vi "LVRT Serial Read LIDAR.vi"(6 "Termination Character (Linefeed)":string="\n", 8 "error in (no error)":errorcluster, 9 "Timeout (ms) (-1: no timeout)":i32=-1, 10 "Bytes to Read":u32, 11 "FPGA Main Ref":T1) -> (0 "error out":errorcluster, 2 "LIDAR":string, 3 "FPGA Main Ref Out":T1)   [LabVIEW 2010]
uses:
  <vilib>/rvi/interface/nirviReadWriteControl/nirviReadWriteControl.xnode
  serial FPGA Main.vi
  FPGA Bitfiles/Athena Brain.lvproj_FPGA Target 2_serial FPGA Main.vi.lvbitx
  serial FPGA main reference type def.ctl
  <vilib>/rvi/errors/niLvFpgaWhatHappensToTopLevelVI.ctl
  <vilib>/rvi/interface/common/niFpgaNodeNameForErrorReporting.ctl
  <vilib>/rvi/errors/niLvFpgaAdjustHostInterfaceError.vi
  <vilib>/RVI Host/nirviSupport.llb/nirviErrorClusterFromErrorCode.vi
panel:
  out "Bytes read so far":u32
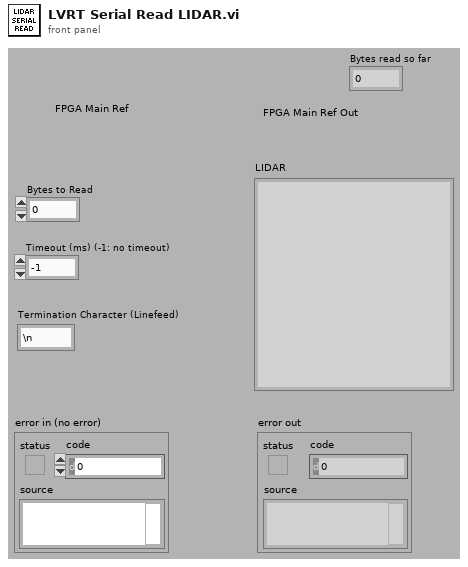
[diagram p1: front panel]
types:
  T1 = typedef "serial FPGA main reference type def.ctl" = refnum<k20>
  T2 = typedef "niFpgaNodeNameForErrorReporting.ctl" = enum16{"Open FPGA VI Reference", "Read/Write Control", "Invoke Method: Abort", "Invoke Method: Acknowledge IRQ", "Invoke Method: Download", "Invoke Method: FIFO.Configure", "Invoke Method: FIFO.Read", "Invoke Method: FIFO.Start", "Invoke Method: FIFO.Stop", "Invoke Method: FIFO.Write", "Invoke Method: Reset", "Invoke Method: Run", "Invoke Method: Wait on IRQ", "Close FPGA VI Reference"}
  T3 = typedef "niLvFpgaWhatHappensToTopLevelVI.ctl" = enum16{"top level VI scripted behind XNode", "top level VI inlined behind XNode"}
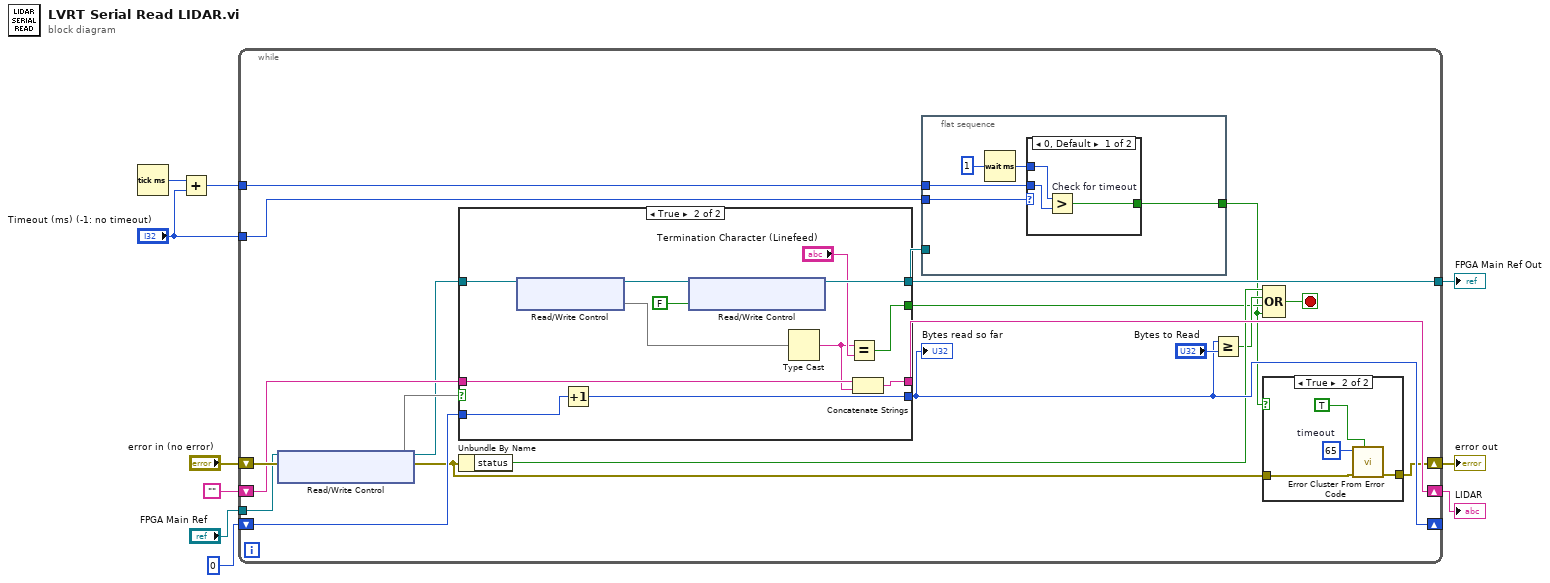
[diagram p0: block diagram]
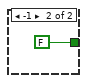
[diagram p3: hidden frame]
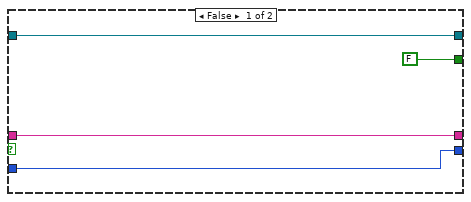
[diagram p4: hidden frame]
diagram:
  n1 = Tick Count (ms)() -> (millisecond timer value=w3:u32)
  n2 = Add(x=w3, y="Timeout (ms) (-1: no timeout)") -> (x+y=w1:u32)
  n3 = while {
    tunnel: "FPGA Main Ref" -> [w23]
    tunnel: [w21] -> w7
    shift-right: [w20] -> _
    shift-left: u32 0 -> [w27]
    shift-right: [w25] -> w4
    shift-left: "" -> [w26]
    shift-right: [w11] -> w9
    shift-left: "error in (no error)" -> [w29]
    tunnel: "Timeout (ms) (-1: no timeout)" -> [w15]
    tunnel: w1 -> [w14]
    stop <- w17 stop-if-true
    n4 = xnode "Read/Write Control"("FPGA VI Reference In"=w23, "error in"=w29) -> ("FPGA VI Reference Out"=w22:T1, "error out"=w12:errorcluster, "LIDAR Read: New Data"=w28)
    n5 = case shown="True" w28 {
      tunnel: [w47 w59] -> w20
      tunnel: w27 -> [w47 w58]
      tunnel: w26 -> [w46 w57]
      tunnel: [w46 w56] -> w25
      tunnel: w22 -> [w45 w54]
      tunnel: [w45 w52] -> w21
      tunnel: [FALSE w49] -> w16
      frame False {
      }
      frame True {
        n6 = xnode "Read/Write Control"("FPGA VI Reference In"=w54) -> ("FPGA VI Reference Out"=w53:T1, "LIDARRead: Char"=w55)  [unwired: 1 in, 1 out]
        n7 = Increment(x=w58) -> (x+1=w59:u32)
        n8 = xnode "Read/Write Control"("FPGA VI Reference In"=w53, "LIDAR Read: New Data"=FALSE ("Data Read")) -> ("FPGA VI Reference Out"=w52:T1)  [unwired: 1 in, 1 out]
        n9 = Type Cast(x=w55) -> (*(type *) &x=w50:string)  [unwired: 1 out]
        n10 = Equal?(x=w50, y="Termination Character (Linefeed)") -> (x = y?=w49:bool)
        n11 = Concatenate Strings(w57, w50) -> (w56:string)
      }
    }
    "Bytes read so far" <- w20
    n12 = Unbundle By Name(w12) -> ("status"=w19:bool)
    n13 = flat-sequence {
      tunnel: w21 -> [_]
      tunnel: [w38] -> w13
      tunnel: w15 -> [w37]
      tunnel: w14 -> [w36]
      frame #0 {
        n14 = Wait (ms)(milliseconds to wait=u32 1) -> (millisecond timer value=w35:u32)
        n15 = case shown="0, Default" w37 {
          tunnel: [w40 FALSE] -> w38
          tunnel: w36 -> [w41 _]
          tunnel: w35 -> [w42 _]
          frame 0, Default {
            n16 = Greater? "Check for timeout"(x=w42, y=w41) -> (0:w40:bool)
          }
          frame -1 {
          }
        }
      }
    }
    n17 = Greater Or Equal?(x=w20, y="Bytes to Read") -> (x >= y?=w18:bool)
    n18 = Compound Arithmetic op=OR(w19, w18, w16, w13) -> (w17:bool)
    n19 = case shown="True" w13 {
      tunnel: w12 -> [w30 w34]
      tunnel: [w30 w33] -> w11
      frame False {
      }
      frame True {
        w32 = 65  # timeout
        n20 = call <vilib>:"Error Cluster From Error Code.vi"("show call chain? (False)"=TRUE, "error in (no error)"=w34, "error code (0)"=w32) -> ("error out"=w33:errorcluster)  [unwired: 6 out]
      }
    }
  }
  "error out" <- w9
  "LIDAR" <- w4
  "FPGA Main Ref Out" <- w7
